vi "LZW.decode.vi"(0 "data":string, 1 "expected data size":i32=10000, 5 "NumberOfStartBits":u8, 11 "error in (no error)":errorcluster) -> (6 "decoded data":i32[](array[numeric]), 15 "error out":errorcluster)   [LabVIEW 2011]
panel:
  out "Array":i32[](array[numeric])
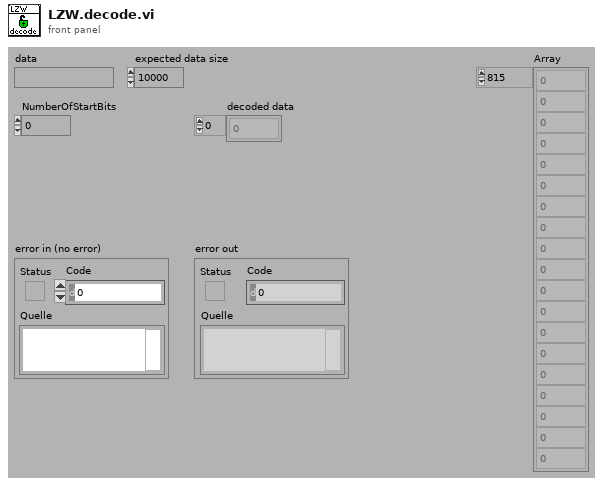
[diagram p1: front panel]
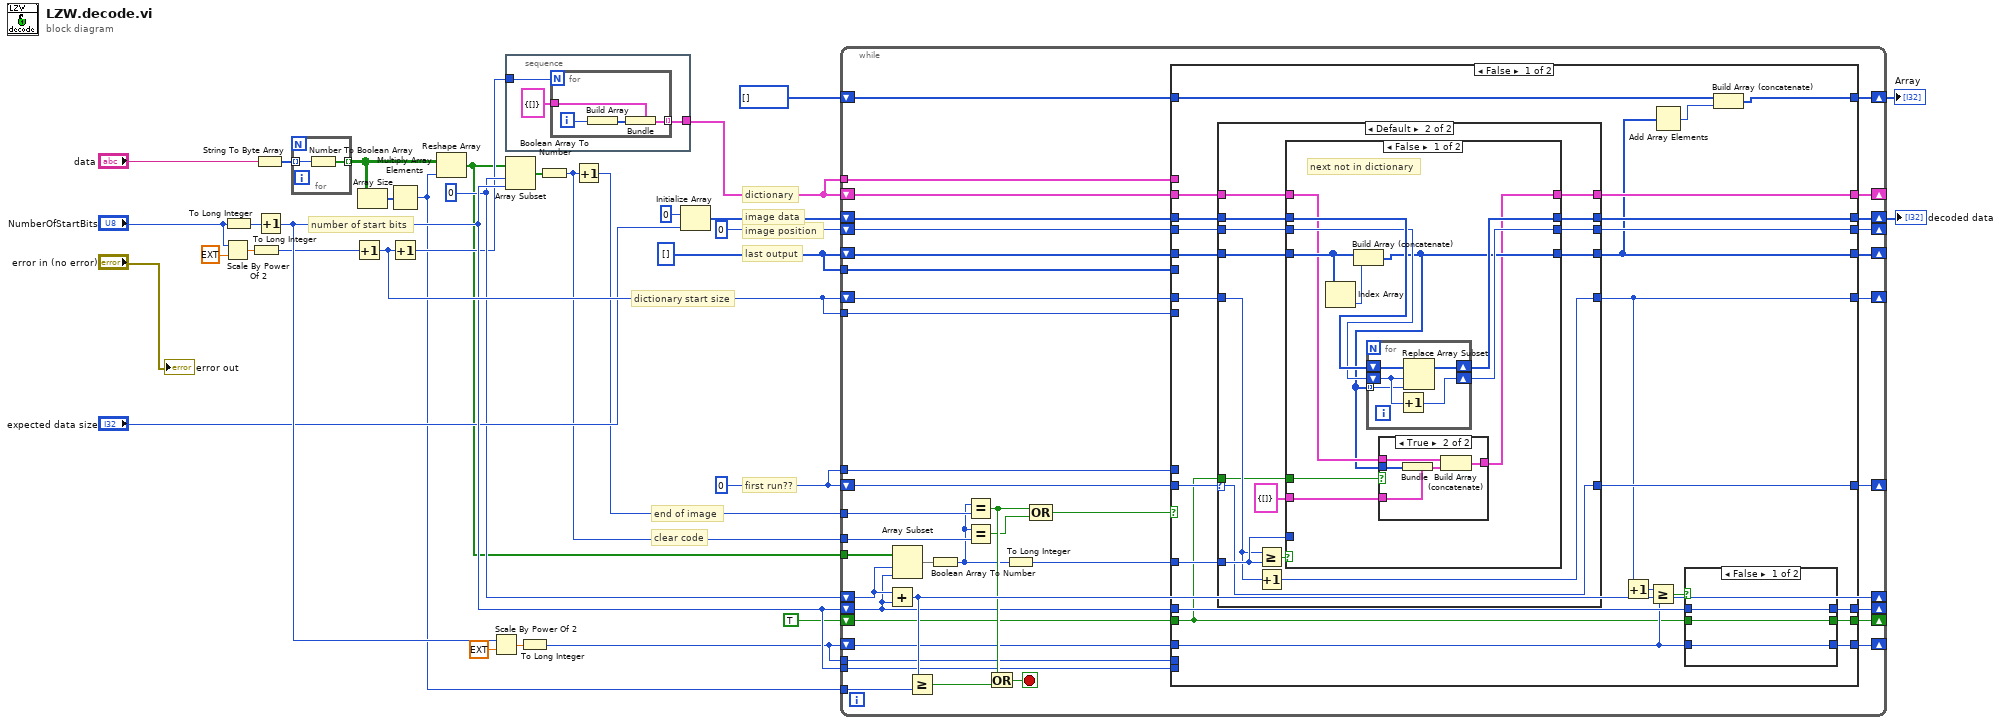
[diagram p0: block diagram]
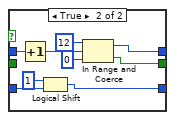
[diagram p2: hidden frame]
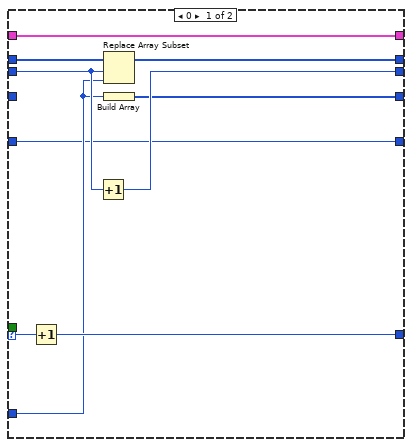
[diagram p3: hidden frame]
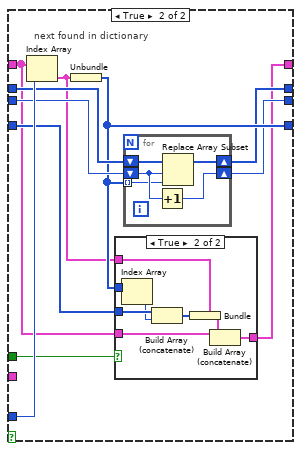
[diagram p5: hidden frame]
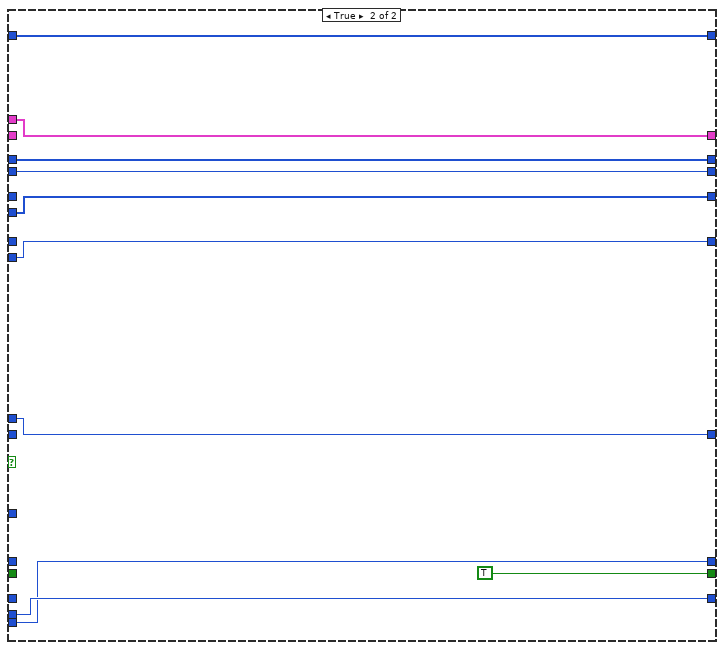
[diagram p7: hidden frame]
diagram:
  w31 = 0
  w24 = i32[] []
  w17 = 0 ("length")
  # "first run??"
  # "last output"
  # "dictionary"
  # "image position"
  # "image data"
  # "dictionary start size"
  # "end of image"
  # "clear code"
  # "number of start bits"
  n1 = Scale By Power Of 2(n="NumberOfStartBits", x=ext 1.0) -> (x*2^n=w8:ext)
  n2 = To Long Integer(number="NumberOfStartBits") -> (32bit integer=w10:i32)
  n3 = To Long Integer(number=w8) -> (32bit integer=w28:i32)
  n4 = String To Byte Array(string="data") -> (unsigned byte array=w15:u8[])
  n5 = Increment(x=w10) -> (x+1=w30:i32)
  n6 = for {
    tunnel: w15 -> [w35] mode=indexing
    tunnel: [w34] -> w5 mode=indexing
    n7 = Number To Boolean Array(number=w35) -> (Boolean array=w34:bool[])
  }
  n8 = Increment(x=w28) -> (x+1=w33:i32)
  n9 = Array Size(array=w5) -> (size(s)=w6:i32[])
  n10 = Multiply Array Elements(1:w6) -> (0:w11:i32)
  n11 = Increment(x=w33) -> (x+1=w16:i32)
  n12 = Reshape Array(w5, w11) -> (w13:bool[])
  n13 = Scale By Power Of 2(n=w30, x=ext 1.0) -> (x*2^n=w26:ext)
  n14 = stacked-sequence {
    tunnel: [w37] -> w25
    tunnel: w16 -> [w36]
    frame #0 {
      n15 = for {
        N: w36 -> [_]
        tunnel: cluster{i32[]} {[]} -> [w40]
        tunnel: [w39] -> w37 mode=indexing
        i -> [w42]
        n16 = Build Array(w42) -> (w41:i32[])
        n17 = Bundle(cluster=w40, w41) -> (w39:cluster{i32[]})
      }
    }
  }
  n18 = Array Subset(array=w13, index=w17, length=w30) -> (w12:bool[])
  n19 = To Long Integer(number=w26) -> (32bit integer=w29:i32)
  n20 = Boolean Array To Number(Boolean array=w12) -> (number=w18:u32)
  n21 = Increment(x=w18) -> (x+1=w19:u32)
  n22 = Initialize Array(0 ("element"), "expected data size") -> (w22:i32[])
  n23 = while {
    tunnel: w13 -> [w81]
    shift-right: [w57] -> _
    shift-left: w30 -> [w59]
    shift-right: [w79] -> _
    shift-left: w17 -> [w80]
    tunnel: w11 -> [w78]
    tunnel: w18 -> [w77]
    tunnel: w19 -> [w76]
    shift-right: [w60] -> _
    shift-left: w33 -> [w61]
    shift-right: [w69] -> w32
    shift-left: w22 -> [w65]
    shift-right: [w68] -> _
    shift-left: 0 ("element") -> [w63]
    shift-right: [w71] -> _
    shift-left: w25 -> [w64]
    shift-right: [w66] -> _
    shift-left: w24 -> [w62]
    tunnel: w25 -> [w70]
    tunnel: w24 -> [w67]
    shift-right: [w56] -> _
    shift-left: w29 -> [w58]
    tunnel: w29 -> [w55]
    tunnel: w30 -> [w54]
    shift-right: [w52] -> _
    shift-left: w31 -> [w53]
    tunnel: w31 -> [w51]
    tunnel: w33 -> [w48]
    shift-right: [w47] -> _
    shift-left: TRUE -> [w46]
    shift-right: [w44] -> w2
    shift-left: i32[] [] -> [w45]
    stop <- w72 stop-if-true
    n24 = Add(x=w80, y=w59) -> (x+y=w79:i32)
    n25 = Array Subset(array=w81, index=w80, length=w59) -> (w82:bool[])
    n26 = Greater Or Equal?(x=w79, y=w78) -> (x >= y?=w73:bool)
    n27 = Boolean Array To Number(Boolean array=w82) -> (number=w50:u32)
    n28 = Equal?(x=w50, y=w76) -> (x = y?=w74:bool)
    n29 = Equal?(x=w50, y=w77) -> (x = y?=w43:bool)
    n30 = Or(x=w74, y=w73) -> (x .or. y?=w72:bool)
    n31 = To Long Integer(number=w50) -> (32bit integer=w49:i32)
    n32 = Compound Arithmetic op=OR(w74, w43) -> (w75:bool)
    n33 = case shown="False" w75 {
      tunnel: w49 -> [w102 _]
      tunnel: [w98 w200] -> w71
      tunnel: w70 -> [_ w200]
      tunnel: [w100 w194] -> w69
      tunnel: [w101 w193] -> w68
      tunnel: w67 -> [_ w199]
      tunnel: [w86 w199] -> w66
      tunnel: w65 -> [w104 w194]
      tunnel: w64 -> [w99 _]
      tunnel: w63 -> [w103 w193]
      tunnel: w62 -> [w89 _]
      tunnel: w61 -> [w97 _]
      tunnel: [w96 w195] -> w60
      tunnel: w59 -> [w93 _]
      tunnel: w58 -> [w90 _]
      tunnel: [w92 w197] -> w57
      tunnel: [w91 w198] -> w56
      tunnel: w55 -> [_ w198]
      tunnel: w54 -> [_ w197]
      tunnel: w53 -> [w106 _]
      tunnel: [w105 w196] -> w52
      tunnel: w51 -> [_ w196]
      tunnel: w48 -> [_ w195]
      tunnel: [w88 TRUE] -> w47
      tunnel: w46 -> [w87 _]
      tunnel: w45 -> [w84 w191]
      tunnel: [w83 w191] -> w44
      frame False {
        n34 = case shown="Default" w106 {
          selector: w106 -> [w128 w130]
          tunnel: [w127 w130] -> w105
          tunnel: w104 -> [w126 w141]
          tunnel: w103 -> [w125 w139]
          tunnel: w102 -> [w121 w137]
          tunnel: [w124 w134] -> w101
          tunnel: [w123 w135] -> w100
          tunnel: w99 -> [w122 w138]
          tunnel: [w122 w133] -> w98
          tunnel: [w120 w136] -> w86
          tunnel: [w119 w143] -> w96
          tunnel: w97 -> [w119 w132]
          tunnel: w89 -> [_ w140]
          tunnel: w87 -> [_ w129]
          frame 0 {
            n35 = Increment(x=w128) -> (x+1=w127:i32)
            n36 = Increment(x=w125) -> (x+1=w124:i32)
            n37 = Replace Array Subset(array=w126, new element=w121, index=w125) -> (w123:i32[])
            n38 = Build Array(w121) -> (w120:i32[])
          }
          frame Default {
            n39 = Greater Or Equal?(x=w132, y=w137) -> (x >= y?=w142:bool)
            n40 = Increment(x=w132) -> (x+1=w143:i32)
            n41 = case shown="False" w142 {
              tunnel: w141 -> [w152 w175]
              tunnel: w140 -> [w154 w170]
              tunnel: w139 -> [w151 w174]
              tunnel: w138 -> [w148 w168]
              tunnel: w137 -> [_ w176]
              tunnel: [w146 w173] -> w136
              tunnel: [w150 w172] -> w135
              tunnel: [w149 w171] -> w134
              tunnel: cluster{i32[]} {[]} -> [w147 _]
              tunnel: [w145 w167] -> w133
              tunnel: w129 -> [w144 w166]
              frame False {
                # "next not in dictionary"
                n42 = Index Array(array=w154) -> (element=w153:i32)  [unwired: 1 in]
                n43 = Build Array (concatenate)(w154, w153) -> (w146:i32[])
                n44 = for {
                  shift-right: [w164] -> w150
                  shift-left: w152 -> [w165]
                  shift-right: [w162] -> w149
                  shift-left: w151 -> [w163]
                  tunnel: w146 -> [w161] mode=indexing
                  n45 = Increment(x=w163) -> (x+1=w162:i32)
                  n46 = Replace Array Subset(array=w165, new element=w161, index=w163) -> (w164:i32[])
                }
                n47 = case shown="True" w144 {
                  tunnel: w148 -> [w155 w160]
                  tunnel: w147 -> [_ w159]
                  tunnel: w146 -> [_ w158]
                  tunnel: [w155 w157] -> w145
                  frame False {
                  }
                  frame True {
                    n48 = Bundle(cluster=w159, w158) -> (w156:cluster{i32[]})
                    n49 = Build Array (concatenate)(w160, w156) -> (w157:cluster{i32[]}[])
                  }
                }
              }
              frame True {
                # "next found in dictionary"
                n50 = Index Array(array=w168, index=w176) -> (element=w169:cluster{i32[]})
                n51 = Unbundle(w169) -> (w173:i32[])
                n52 = case shown="True" w166 {
                  tunnel: w173 -> [_ w185]
                  tunnel: w170 -> [_ w184]
                  tunnel: w169 -> [_ w182]
                  tunnel: w168 -> [w177 w180]
                  tunnel: [w177 w178] -> w167
                  frame False {
                  }
                  frame True {
                    n53 = Index Array(array=w185) -> (element=w183:i32)  [unwired: 1 in]
                    n54 = Build Array (concatenate)(w184, w183) -> (w181:i32[])
                    n55 = Bundle(cluster=w182, w181) -> (w179:cluster{i32[]})
                    n56 = Build Array (concatenate)(w180, w179) -> (w178:cluster{i32[]}[])
                  }
                }
                n57 = for {
                  shift-right: [w189] -> w172
                  shift-left: w175 -> [w190]
                  shift-right: [w187] -> w171
                  shift-left: w174 -> [w188]
                  tunnel: w173 -> [w186] mode=indexing
                  n58 = Increment(x=w188) -> (x+1=w187:i32)
                  n59 = Replace Array Subset(array=w190, new element=w186, index=w188) -> (w189:i32[])
                }
              }
            }
          }
        }
        n60 = Increment(x=w96) -> (x+1=w95:i32)
        n61 = Greater Or Equal?(x=w95, y=w90) -> (x >= y?=w94:bool)
        n62 = Add Array Elements(numeric array=w86) -> (sum=w85:i32)
        n63 = case shown="False" w94 {
          tunnel: w93 -> [w109 w118]
          tunnel: [w109 w111] -> w92
          tunnel: [w108 w115] -> w91
          tunnel: w90 -> [w108 w117]
          tunnel: [w107 w110] -> w88
          tunnel: w87 -> [w107 _]
          frame False {
          }
          frame True {
            n64 = Increment(x=w118) -> (x+1=w112:i32)
            n65 = Logical Shift(y=1, x=w117) -> (x << y=w115:i32)
            n66 = In Range and Coerce(upper limit=12, x=w112, lower limit=0) -> (coerced(x)=w111:i32, In Range?=w110:bool)
          }
        }
        n67 = Build Array (concatenate)(w84, w85) -> (w83:i32[])
      }
      frame True {
      }
    }
  }
  "decoded data" <- w32
  "Array" <- w2
  "error out" <- "error in (no error)"
